vi "Test_API_DelayedShutdown_PostShutdownEventsCaptured.vi"(8 "error in (no error)":errorcluster, 11 "TestCase in":refnum<class "TestComposedLog.lvclass">) -> (0 "error out":errorcluster, 3 "TestCase out":refnum<class "TestComposedLog.lvclass">)   [LabVIEW 2019, in "TestComposedLog.lvclass"]
uses:
  TestComposedLog.lvclass
  Source/Composed Log/Types/Log Level.ctl
  Source/Composed Log/LoggerReference/LoggerReference.lvclass/LoggerReference.ctl
  Source/LVQueue Sink/LVQueue Sink.lvclass/LVQueue Sink.ctl
  d49e4f2a-1326-4cbd-a2c1-f46e8011f9e4.vi
  d49e4f2a-1326-4cbd-a2c1-f46e8011f9e4.vi/ce85b877-45d5-4a3f-b4ab-07c873b82621.vi
  Source/Composed Log/LoggerReference/Return Aggregate Queues.vi
  Source/Composed Log/LoggerReference/Add Aggregate Log.vi
  d49e4f2a-1326-4cbd-a2c1-f46e8011f9e4.vi/ce85b877-45d5-4a3f-b4ab-07c873b82621.vi/ed750467-268e-4c99-9917-96796c87ddfd.vi
  Source/Composed Log/LoggerReference/Log.vi
  Source/Composed Log/LoggerReference/Get Valid Event Time.vi
  Source/Composed Log/LoggerReference/Send Add Sink.vi
  Source/Composed Log/LoggerReference/Remove Stale Logs.vi
  Source/LVQueue Sink/LVQueue Sink.lvclass
  C:/CS/Log/Source/Composed Log/Log Sink/Log Sink.lvclass
  Source/Composed Log/Application Logger/Launch Worker Loop.vi
  Source/Composed Log/LoggerReference/Initialize Logger Instance.vi
  Source/Composed Log/Singleton Event Log/Logger Queue FGV.vi
  Source/Composed Log/IErrorFormat/IErrorFormat.lvclass
  Source/Composed Log/LoggerReference/LoggerReference.lvclass
  Source/Composed Log/Log Sink/Log Sink.lvclass
  <vilib>/addons/_JKI Toolkits/VI Tester/TestCase.llb/TestCase.lvclass
  Source/Composed Log/Singleton Event Log/Singleton Event Log.lvlib
  Source/Composed Log/Composed Log.lvlib
  C:/Program Files (x86)/National Instruments/LabVIEW 2019/vi.lib/addons/_JKI Toolkits/VI Tester/TestCase.llb/TestCase.lvclass
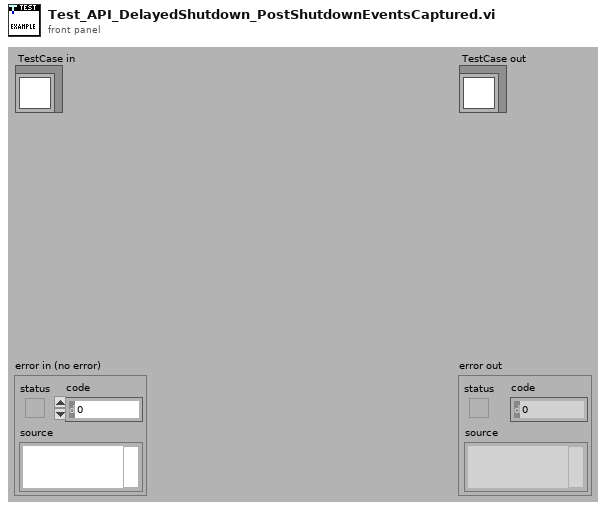
[diagram p1: front panel]
types:
  T1 = typedef "Composed Log.lvlib/Log Level.ctl" = enum16{"Debug", "Info", "Warning", "Error", "Critical"}
  T2 = typedef "Composed Log.lvlib/Log Packet.ctl" = cluster{"Data To Log":string, "Source":string, "Event Level":T1, "Event Time":timestamp}
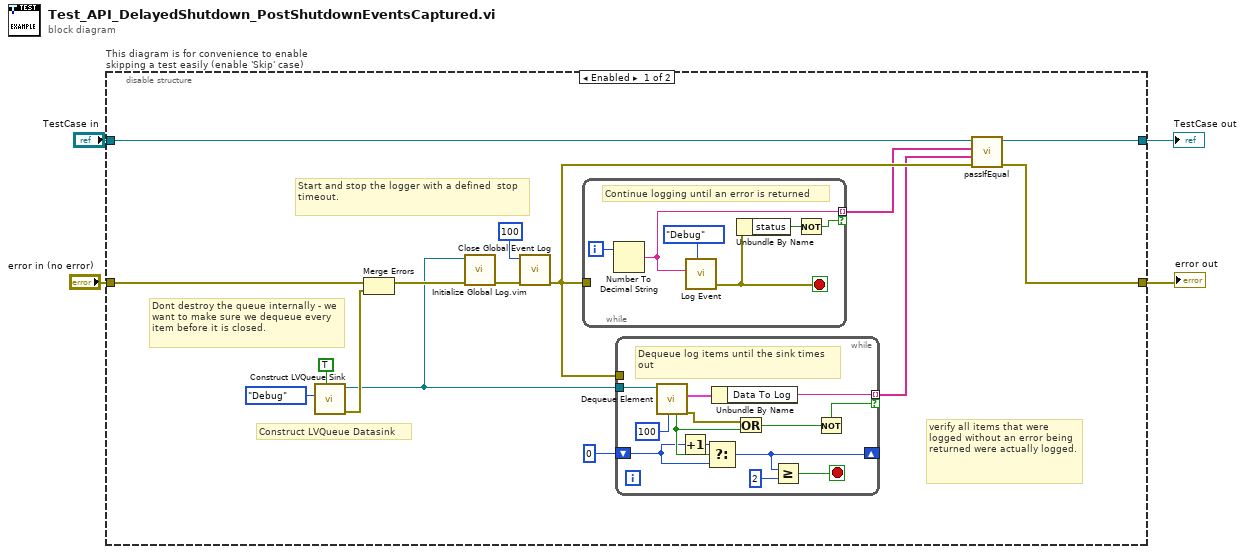
[diagram p0: block diagram]
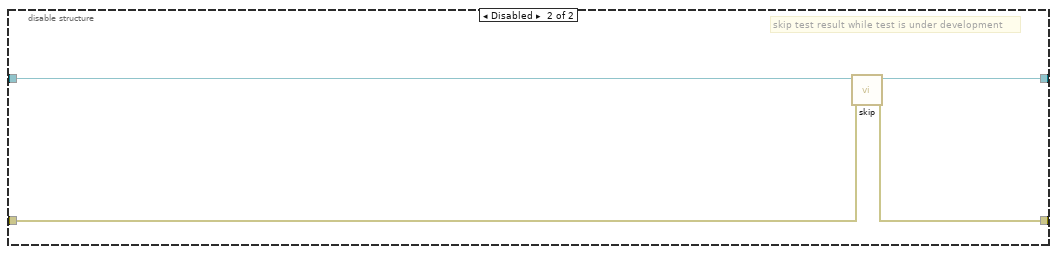
[diagram p2: hidden frame]
diagram:
  n1 = disable-structure "This diagram is for convenience to enable skipping a test easily (enable 'Skip' case)" shown="Enabled" {
    disable-tunnel: "TestCase in" -> [w17 w42]
    disable-tunnel: [w18 w40] -> w1
    disable-tunnel: [w16 w41] -> w3
    disable-tunnel: "error in (no error)" -> [w19 w39]
    frame Enabled {
      # "Dont destroy the queue internally - we want to make sure we dequeue every item before it is closed."
      # "verify all items that were logged without an error being returned were actually logged."
      # "Construct LVQueue Datasink"
      # "Start and stop the logger with a defined  stop timeout."
      n2 = call "Construct LVQueue Sink.vi"("User Shutdown? (F)"=TRUE, "LogLevel"=Log_Level."Debug") -> ("error out"=w13:errorcluster, "LVQueue Sink out"=w8:refnum<class "LVQueue Sink.lvclass">)  [unwired: 8 in]
      n3 = Merge Errors(w19, w13) -> (w14:errorcluster)
      n4 = call "Initialize Global Log.vim"("error in (no error)"=w14, "Log Sink(s)"=w8) -> ("error out"=w12:errorcluster)  [unwired: 8 in, 1 out]
      n5 = call "Close Global Event Log.vi"("error in (no error)"=w12, "Deferred Close Time (0 ms)"=u32 100 ("Deferred Close Time (ms)")) -> ("error out"=w10:errorcluster)  [unwired: 9 in]
      n6 = while {
        tunnel: w10 -> [_]
        tunnel: [w34] -> w5 mode=indexing if=w36
        i -> [w38]
        stop <- w35 stop-if-true
        # "Continue logging until an error is returned"
        n7 = Number To Decimal String(number=w38) -> (decimal integer string=w34:string)  [unwired: 1 in]
        n8 = call "Log Event.vi"("Event Level"=Log_Level."Debug", "Data To Log"=w34) -> ("error out"=w35:errorcluster)  [unwired: 9 in]
        n9 = Unbundle By Name(w35) -> ("status"=w37:bool)
        n10 = Not(x=w37) -> (.not. x?=w36:bool)
      }
      n11 = while {
        tunnel: w8 -> [w32]
        tunnel: [w29] -> w7 mode=indexing if=w27
        tunnel: w10 -> [_]
        shift-right: [w22] -> _
        shift-left: 0 -> [w23]
        stop <- w20 stop-if-true
        # "Dequeue log items until the sink times out"
        n12 = call "Dequeue Element.vi"("timeout in ms (-1)"=100, "LVQueue Sink in"=w32) -> ("error out"=w28:errorcluster, "Log Packet"=w30:T2, "Timed Out?"=w25:bool)  [unwired: 6 in, 1 out]
        n13 = Increment(x=w23) -> (x+1=w24:i32)
        n14 = Select(t=w24, s=w25, f=w23) -> (s? t:f=w22:i32)
        n15 = Unbundle By Name(w30) -> ("Data To Log"=w29:string)
        n16 = Or(x=w28, y=w25) -> (x .or. y?=w26:bool)
        n17 = Greater Or Equal?(x=w22, y=2) -> (x >= y?=w20:bool)
        n18 = Not(x=w26) -> (.not. x?=w27:bool)
      }
      n19 = call-dynamic "passIfEqual.vi"("error in (no error)"=w10, "y"=w7, "x"=w5, "TestCase in"=w17) -> ("error out"=w16:errorcluster, "TestCase out"=w18:refnum<class "TestComposedLog.lvclass">)  [unwired: 6 in]
    }
    frame Disabled {
      # "skip test result while test is under development"
      n20 = call <vilib>:"skip.vi"("error in (no error)"=w39, "TestCase in"=w42) -> ("error out"=w41:errorcluster, "TestCase out"=w40:refnum<class "TestComposedLog.lvclass">)  [unwired: 8 in]
    }
  }
  "error out" <- w3
  "TestCase out" <- w1
